vi "Is Project SourceOnly.vi"(10 "Project Refnum":refnum<vi>) -> (2 "Is SourceOnly":bool)   [LabVIEW 2020]
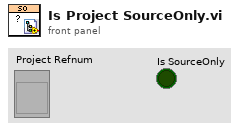
[diagram p1: front panel]
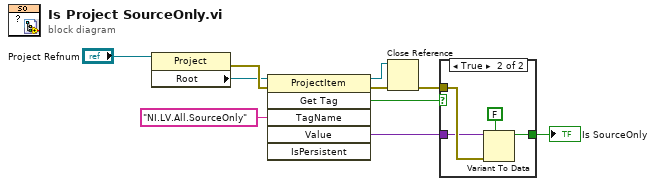
[diagram p0: block diagram]
diagram:
  n1 = property class="Project"(reference="Project Refnum") -> (error out=w10:errorcluster, "Root"=w6:refnum<vi>)  [unwired: 1 in, 1 out]
  n2 = invoke class="ProjectItem" method="Get Tag"(reference=w6, error in=w10, "TagName"="NI.LV.All.SourceOnly" ("Tag Name")) -> (reference out=w1:refnum<vi>, error out=w9:errorcluster, "GetTag"=w4:bool, "Value"=w3:variant)  [unwired: 3 in, 2 out]
  n3 = Close Reference(reference=w1, error in (no error)=w9) -> (error out=w8:errorcluster)
  n4 = case shown="True" w4 {
    tunnel: w3 -> [_ w13]
    tunnel: w8 -> [_ w14]
    tunnel: [_ w11] -> w2
    frame False {
    }
    frame True {
      n5 = Variant To Data(error in=w14, type=FALSE, Variant=w13) -> (data=w11:bool)  [unwired: 1 out]
    }
  }
  "Is SourceOnly" <- w2
